vi "Measurement Logic.vi"() -> ()   [LabVIEW 2021, in "Single Tone Power Sweep.lvlib"]
uses:
  Single Tone Power Sweep.lvlib
  Measurement Configuration.ctl
  shared/controls/digital output level units.ctl
  shared/controls/weighting filter.ctl
  shared/controls/highpass filter.ctl
  shared/controls/lowpass filter.ctl
  shared/controls/units - snr.ctl
  shared/controls/units - ratio.ctl
  shared/controls/power measurement method.ctl
  Measurement Results.ctl
  <vilib>/MeasurementLink/MeasurementLink Measurement Server/Measure Call Context/Measure Call Context.lvclass
  <instrlib>/niDCPower/nidcpower.llb/niDCPower Source Mode.ctl
  <instrlib>/niDCPower/nidcpower.llb/niDCPower Output Function.ctl
  <instrlib>/niDMM/nidmm.llb/niDMM Function.ctl
  <instrlib>/niDMM/nidmm.llb/niDMM Resolution in Digits.ctl
  <vilib>/Analysis/1siggen.llb/Ramp Pattern by Samples.vi
  <instrlib>/niDMM/nidmm.llb/niDMM Configure Measurement Digits.vi
  <vilib>/Analysis/NI_AALBase.lvlib
  shared/controls/audio controls.lvlib
panel:
  out "XY Graph":cluster{"Array":dbl[], "Array":dbl[]}(graph)
  out "Spectrum":cluster{"x0":dbl, "dx":dbl, "magnitude":dbl[]}[](graph)
  out "Waveform Graph":waveform(dbl)[](graph)
  out "measure call context out":refnum<class "Measure Call Context.lvclass">
  in  "measure call context in":refnum<class "Measure Call Context.lvclass">
  out "measurement results":T1={"channel names"=[], "SNR"=[], "THD+N"=[], "THD"=[], "power supply voltage (V)"=[], "power supply current (A)"=[], "input power (W)"=[], "total output power (W)"=[], "power loss (W)"=[], "efficiency (%)"=[], "wfm - t0"=0.0, "wfm - dt"=1.9531249997269942e-05, "wfm - data"=array[12800 elements], "fft - f0"=0.0, "fft - df"=4.000000000559116, "fft - data"=array[6400 elements]}
  in  "measurement configuration":T2={"digital serial cfg file"="", "digital channel list"="7821\\PCMo 8", "master clock channel list"="7821\\PCMo 0", "output level start"=10.0, "output level stop"=60.0, "output sweep number of steps"=5, "output level units"=enum."% FS", "output range (pk-pk)"=15.0, "load impedance"=4.0, "signal phase"=0.0, "acq sampling rate"=51200.0, "min measurement cycles"=20, "min measurement time (s)"=0.1, "min settling cycles"=0, "min settling time (s)"=0.005, "acq channel"="PXI1Slot4/ai0", "band start"=20.0, "band stop"=20000.0, "weighting filter"=enum."Linear", "highpass filter"=enum."DC", "lowpass filter"=enum."No filter", "SNR units"=enum."dB", "THD+N units"=enum."dB", "THD units"=enum."dB", "gain units"=enum."dB", "power measurement method"=enum."DMM", "power measurement resource"="PXI1Slot9", "power supply voltage"=14.4, "power supply current limit"=1.2, "sense resistor (Ohms)"=0.01} {"band start" format="%0.2f"; "acq sampling rate" format="%0.2f"; "signal phase" format="%#_6p"}
  out "error out":errorcluster
  in  "error in":errorcluster
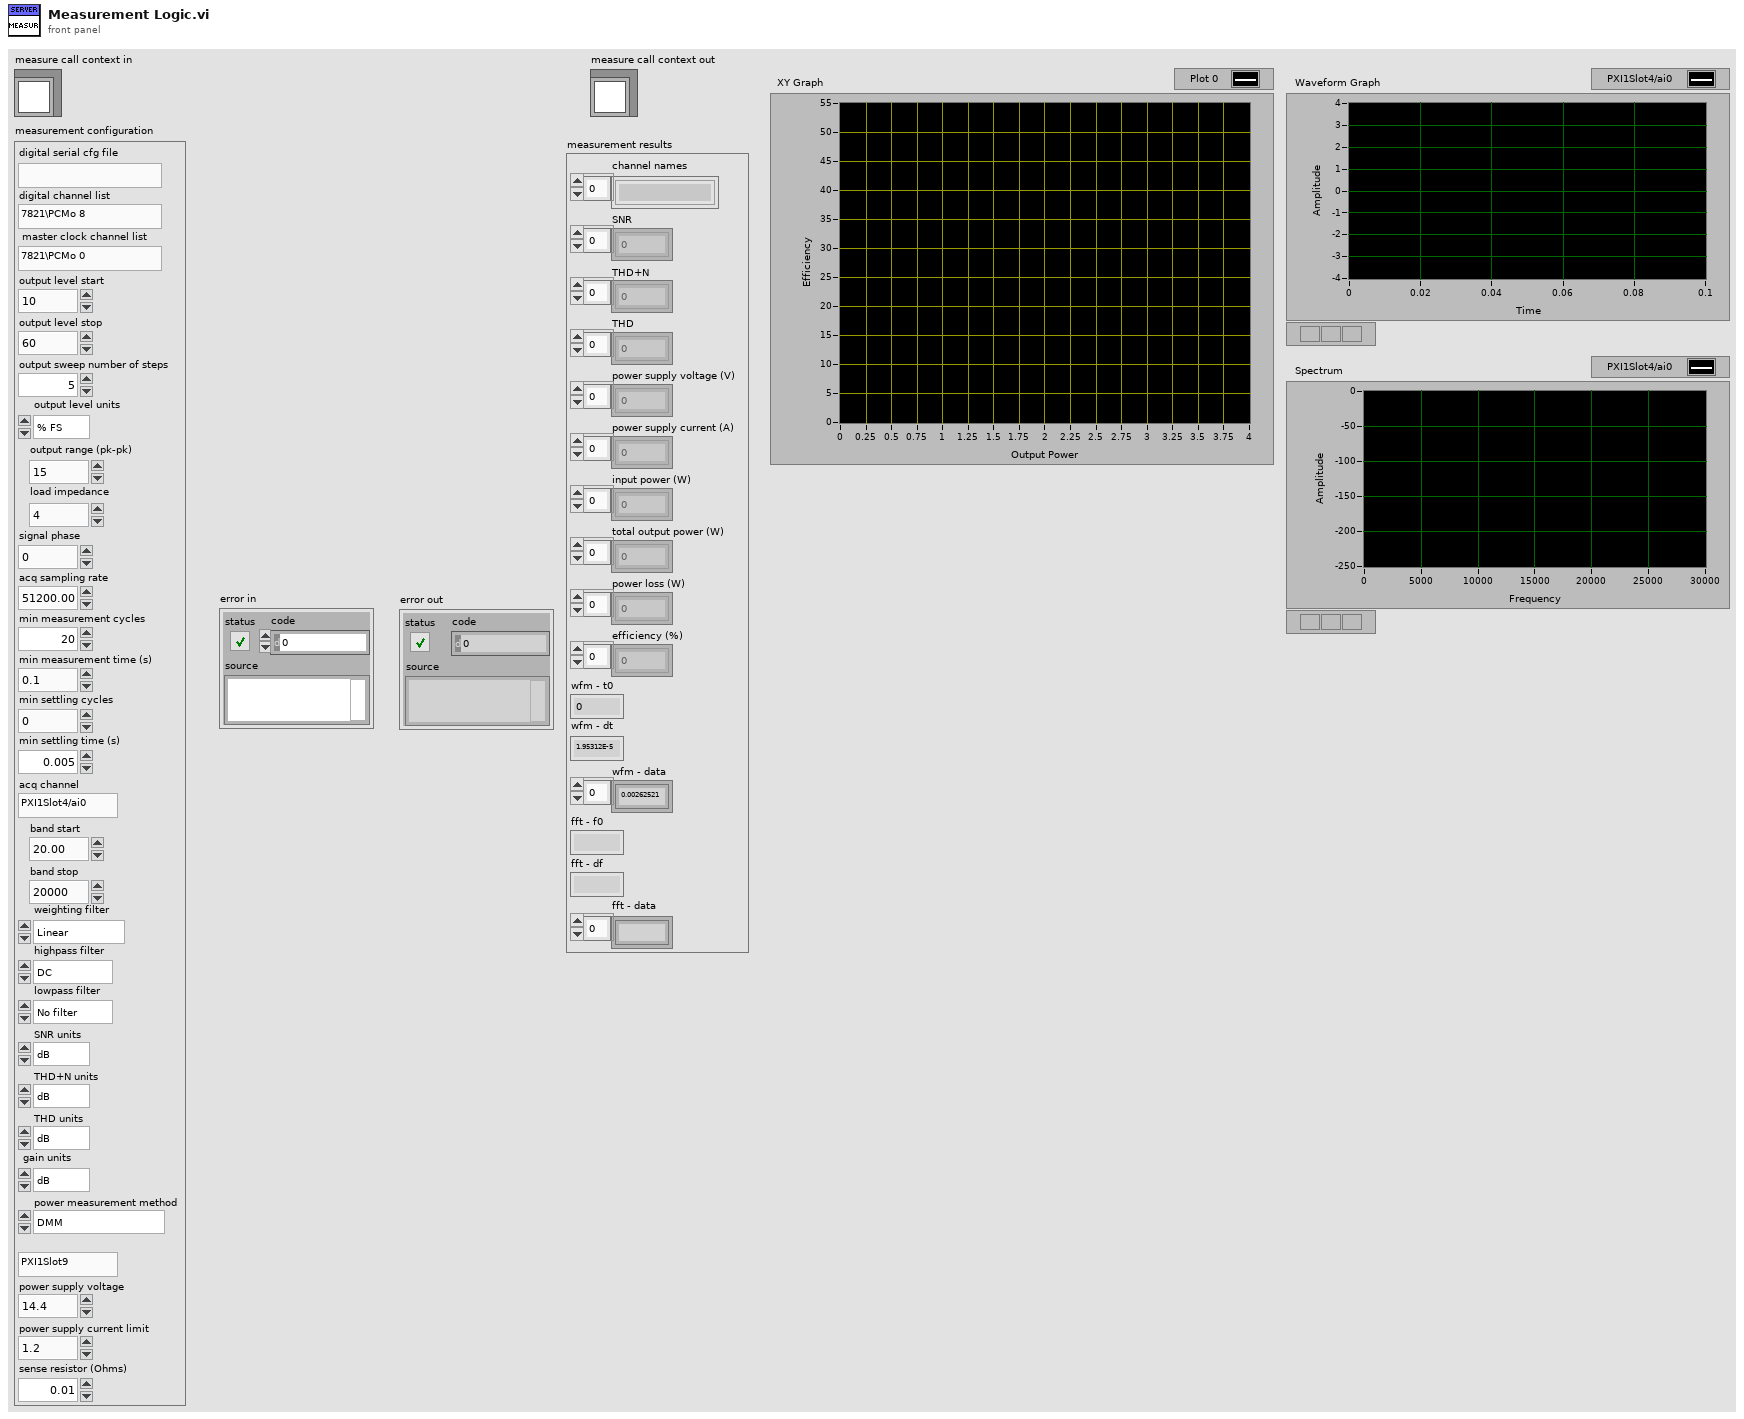
[diagram p1: front panel]
types:
  T1 = typedef "Single Tone Power Sweep.lvlib/Measurement Results.ctl" = cluster{"channel names":string[], "SNR":dbl[], "THD+N":dbl[], "THD":dbl[], "power supply voltage (V)":dbl[], "power supply current (A)":dbl[], "input power (W)":dbl[], "total output power (W)":dbl[], "power loss (W)":dbl[], "efficiency (%)":dbl[], "wfm - t0":dbl, "wfm - dt":dbl, "wfm - data":dbl[], "fft - f0":dbl, "fft - df":dbl, "fft - data":dbl[]}
  T2 = typedef "Single Tone Power Sweep.lvlib/Measurement Configuration.ctl" = cluster{"digital serial cfg file":string, "digital channel list":string, "master clock channel list":string, "output level start":dbl, "output level stop":dbl, "output sweep number of steps":u32, "output level units":T3, "output range (pk-pk)":dbl, "load impedance":dbl, "signal phase":dbl, "acq sampling rate":dbl, "min measurement cycles":u32, "min measurement time (s)":dbl, "min settling cycles":u32, "min settling time (s)":dbl, "acq channel":string, "band start":dbl, "band stop":dbl, "weighting filter":T4, "highpass filter":T5, "lowpass filter":T6, "SNR units":T7, "THD+N units":T8, "THD units":T8, "gain units":T8, "power measurement method":T9, "power measurement resource":string, "power supply voltage":dbl, "power supply current limit":dbl, "sense resistor (Ohms)":dbl}
  T3 = typedef "audio controls.lvlib/digital output level units.ctl" = enum32{"% FS", "dBFS", "V"}
  T4 = typedef "weighting filter.ctl" = enum32{"Linear", "A-weighting", "B-weighting", "C-weighting"}
  T5 = typedef "highpass filter.ctl" = enum32{"DC", "AC"}
  T6 = typedef "lowpass filter.ctl" = enum32{"No filter", "AES17 20kHz", "AES17 40kHz"}
  T7 = typedef "audio controls.lvlib/units - snr.ctl" = enum32{"dB", "x/y"}
  T8 = typedef "audio controls.lvlib/units - ratio.ctl" = enum32{"dB", "%", "x/y"}
  T9 = typedef "power measurement method.ctl" = enum32{"SMU", "DMM"}
  T10 = typedef "niDMM Function.ctl" = enum16{"DC Volts", "AC Volts", "DC Current", "AC Current", "2-wire Resistance", "4-wire Resistance", "Diode", "Frequency", "Period", "AC Volts DC Coupled", "Capacitance", "Inductance", "Temperature"}
  T11 = typedef "niDCPower Output Function.ctl" = i32
  T12 = typedef "niDCPower Source Mode.ctl" = i32
  T13 = typedef "niDMM Resolution in Digits.ctl" = dbl
  T14 = typedef "single tone measurement settings (HW).ctl" = cluster{"digital channel list":string, "frame clock rate":dbl, "number of channels":u32, "channel length":u32, "bit depth":u32, "data justification":T15, "endianness":T16, "bit clock edge sync":T17, "frame sync edge for channel 0":T17, "channel 0 offset":u32, "master clock channel list":string, "master clock rate":dbl, "enable dither":bool, "logic level":T18, "signal frequency":dbl, "output level":dbl, "output level units":T3, "output range (pk-pk)":dbl, "load impedance":dbl, "signal phase":dbl, "acq sampling rate":dbl, "min measurement cycles":u32, "min measurement time (s)":dbl, "min settling cycles":u32, "min settling time (s)":dbl, "acq channel":string, "band start":dbl, "band stop":dbl, "weighting filter":T4, "highpass filter":T5, "lowpass filter":T6, "SNR units":T7, "THD+N units":T8, "THD units":T8, "gain units":T8}
  T15 = typedef "data justification.ctl" = enum32{"Left Justified", "Right Justified"}
  T16 = typedef "endianness.ctl" = enum32{"MSB First", "LSB First"}
  T17 = typedef "digital edge.ctl" = enum32{"Rising", "Falling"}
  T18 = typedef "logic level.ctl" = enum32{"3.3 V", "1.8 V", "1.2 V"}
  T19 = typedef "PCM tasks.ctl" = cluster{"PCM output task":T20, "PCM output task-clock":T20}
  T20 = typedef "PDM Acquisition Class Library.lvlib/PCM Output Task.lvclass/PCM Output Task DVR.ctl" = refnum<data-value>
  T21 = typedef "audio controls.lvlib/single tone audio measurements.ctl" = cluster{"channel":string, "frequency (Hz)":dbl, "amplitude (Vrms)":dbl, "amplitude (dBFS)":dbl, "phase (deg)":dbl, "SNR":dbl, "THD+N":dbl, "THD":dbl, "dynamic range (dB)":dbl, "gain":dbl, "SFDR (dBc)":dbl}
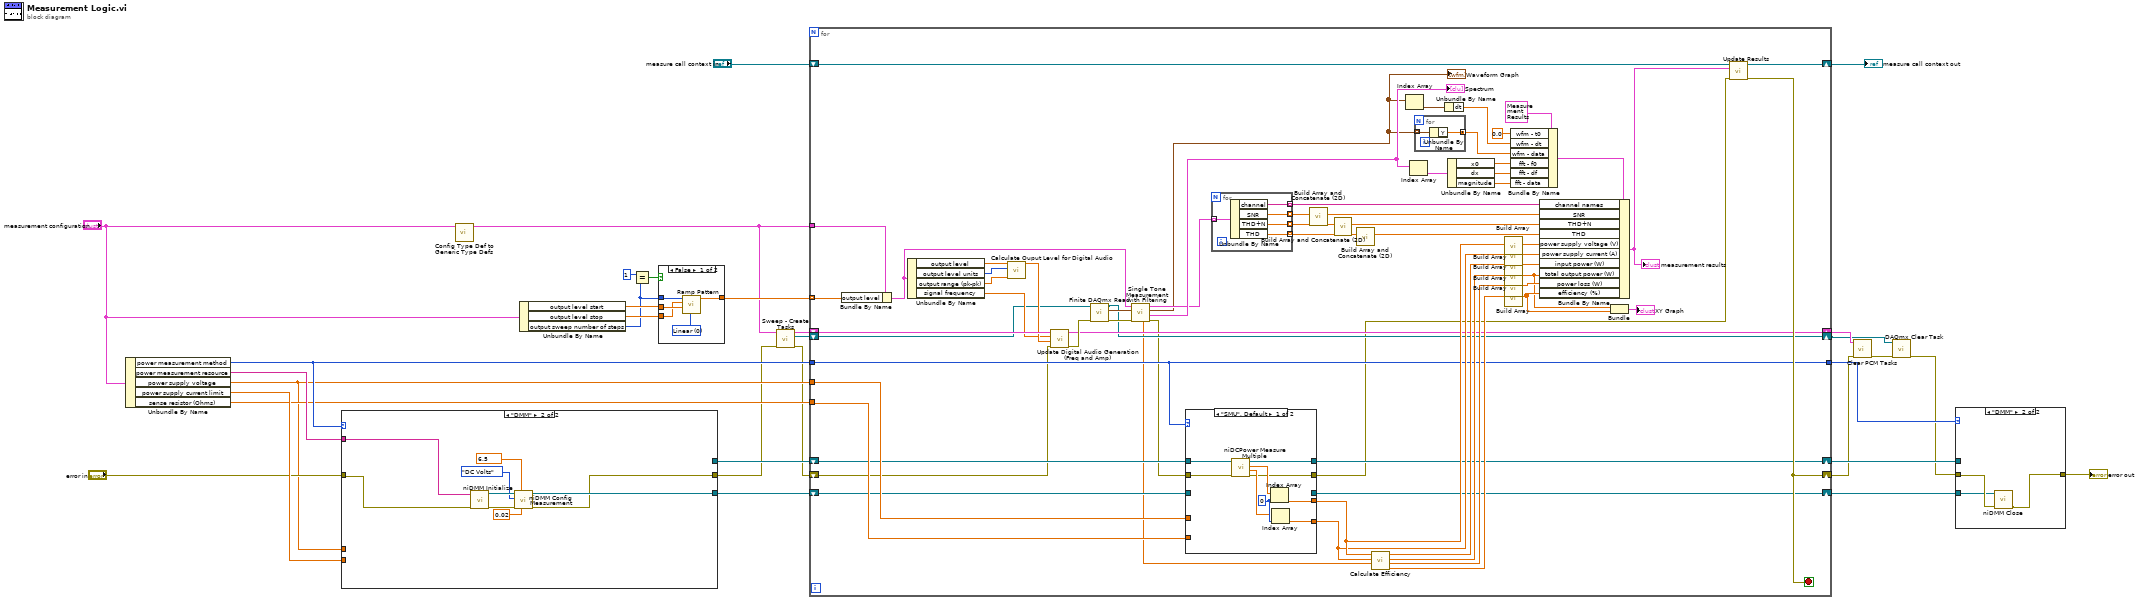
[diagram p0: block diagram]
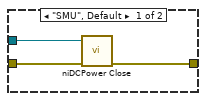
[diagram p2: hidden frame]
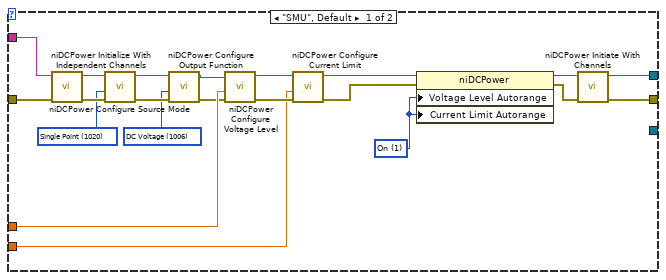
[diagram p3: hidden frame]
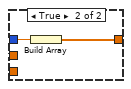
[diagram p4: hidden frame]
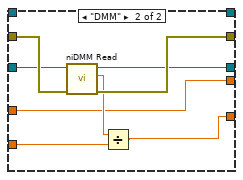
[diagram p5: hidden frame]
diagram:
  n1 = Unbundle By Name("measurement configuration") -> ("power measurement method"=w20:T9, "power measurement resource"=w23:string, "power supply voltage"=w18:dbl, "power supply current limit"=w22:dbl, "sense resistor (Ohms)"=w19:dbl)
  n2 = case shown="\"DMM\"" w20 {
    tunnel: w18 -> [w50 _]
    tunnel: w22 -> [w49 _]
    tunnel: [w35 _] -> w11
    tunnel: [w34 w57] -> w10
    tunnel: "error in" -> [w33 w61]
    tunnel: [_ w58] -> w12
    tunnel: w23 -> [w32 w53]
    frame "SMU", Default {
      w36 = 1 items=["Off", "On"] ("Source:DC Voltage:Current Limit Autorange")
      w37 = T11 1006 items=["DC Voltage"=1006, "DC Current"=1007, "Pulse Voltage"=1049, "Pulse Current"=1050] ("output function")
      w44 = T12 1020 items=["Single Point"=1020, "Sequence"=1021] ("source mode")
      n3 = call <instrlib>:"niDCPower Initialize With Independent Channels.vi"("error in (no error)"=w33, "resource name"=w32) -> ("error out"=w48:errorcluster, "instrument handle out"=w47:refnum<k15>)  [unwired: 8 in]
      n4 = call <instrlib>:"niDCPower Configure Source Mode.vi"("error in (no error)"=w48, "source mode"=w44, "instrument handle"=w47) -> ("error out"=w46:errorcluster, "instrument handle out"=w45:refnum<k15>)  [unwired: 7 out]
      n5 = call <instrlib>:"niDCPower Configure Output Function.vi"("error in (no error)"=w46, "output function"=w37, "instrument handle"=w45) -> ("error out"=w38:errorcluster, "instrument handle out"=w39:refnum<k15>)  [unwired: 1 in, 6 out]
      n6 = call <instrlib>:"niDCPower Configure Voltage Level.vi"("error in (no error)"=w38, "voltage level"=w50, "instrument handle"=w39) -> ("error out"=w51:errorcluster, "instrument handle out"=w52:refnum<k15>)  [unwired: 1 in, 6 out]
      n7 = call <instrlib>:"niDCPower Configure Current Limit.vi"("error in (no error)"=w51, "current limit"=w49, "instrument handle"=w52) -> ("error out"=w40:errorcluster, "instrument handle out"=w43:refnum<k15>)  [unwired: 2 in, 5 out]
      n8 = property class="niDCPower"(reference=w43, error in=w40, "Voltage Level Autorange"=w36, "Current Limit Autorange"=w36) -> (reference out=w42:refnum<k15>, error out=w41:errorcluster)
      n9 = call <instrlib>:"niDCPower Initiate With Channels.vi"("error in (no error)"=w41, "instrument handle"=w42) -> ("error out"=w34:errorcluster, "instrument handle out"=w35:refnum<k15>)  [unwired: 8 in]
    }
    frame "DMM" {
      w55 = T13 6.5 items=["3 1/2"=3.5, "4 1/2"=4.5, "5 1/2"=5.5, "6 1/2"=6.5, "7 1/2"=7.5] ("Resolution in Digits")
      n10 = call <instrlib>:"niDMM Initialize.vi"("error in (no error)"=w61, "Instrument Descriptor"=w53) -> ("error out"=w60:errorcluster, "instrument handle out"=w59:refnum<k15>)  [unwired: 8 in]
      n11 = call-poly <instrlib>:"niDMM Config Measurement.vi"("Range"=0.02, "Resolution in Digits"=w55, "error in (no error)"=w60, "Function"=niDMM_Function."DC Volts", "instrument handle"=w59) -> ("error out"=w57:errorcluster, "instrument handle out"=w58:refnum<k15>)  [unwired: 5 in]
    }
  }
  n12 = call "Config Type Def to Generic Type Defs.vi"("measurement configuration"="measurement configuration") -> ("single tone settings"=w9:T14)  [unwired: 9 in, 1 out]
  n13 = Unbundle By Name("measurement configuration") -> ("output level start"=w31:dbl, "output level stop"=w30:dbl, "output sweep number of steps"=w26:u32)
  n14 = Equal?(x=u32 1, y=w26) -> (x = y?=w27:bool)
  n15 = case shown="False" w27 {
    tunnel: w31 -> [w66 w68]
    tunnel: w30 -> [w65 _]
    tunnel: w26 -> [w64 _]
    tunnel: [w63 w67] -> w29
    frame False {
      w62 = u16 0 items=["Linear", "Logarithmic"] ("type")
      n16 = call-poly <vilib>:"Ramp Pattern.vi"("type"=w62, "start"=w66, "end"=w65, "samples"=w64) -> ("Ramp Pattern"=w63:dbl[])  [unwired: 6 in, 1 out]
    }
    frame True {
      n17 = Build Array(w68) -> (w67:dbl[])
    }
  }
  n18 = call "Sweep - Create Tasks.vi"("error in (no error)"=w10, "measurement configuration"=w9) -> ("error out"=w6:errorcluster, "DAQmx task"=w7:refnum<k21>, "PCM tasks"=w8:T19)  [unwired: 7 in]
  n19 = for {
    tunnel: w29 -> [w106] mode=indexing
    shift-right: [w105] -> w2
    shift-left: w6 -> [w81]
    shift-right: [w131] -> w28
    shift-left: "measure call context in" -> [w130]
    tunnel: w20 -> [w104]
    tunnel: w19 -> [w121]
    tunnel: w18 -> [w120]
    tunnel: w9 -> [w107]
    tunnel: [w104] -> w15
    shift-right: [w103] -> w14
    shift-left: w11 -> [w97]
    shift-right: [w102] -> w13
    shift-left: w12 -> [w98]
    shift-right: [w89] -> w4
    shift-left: w8 -> [w90]
    shift-right: [w85] -> w3
    shift-left: w7 -> [w84]
    stop <- w105 stop-if-true
    n20 = Bundle By Name(cluster=w107, "output level"=w106) -> (w86:T14)
    n21 = Unbundle By Name(w86) -> ("output level"=w96:dbl, "output level units"=w95:T3, "output range (pk-pk)"=w94:dbl, "signal frequency"=w87:dbl)
    n22 = call "Calculate Ouput Level for Digital Audio.vi"("output range (pk-pk)"=w94, "digital output level units"=w95, "output level"=w96) -> ("gain"=w88:dbl)  [unwired: 7 in, 1 out]
    n23 = call "Update Digital Audio Generation (Freq and Amp).vi"("error in (no error)"=w81, "gain"=w88, "frequency"=w87, "PCM tasks"=w90) -> ("error out"=w93:errorcluster, "PCM tasks"=w89:T19)  [unwired: 6 in]
    n24 = call "Finite DAQmx Read.vi"("error in (no error)"=w93, "task/channels in"=w84) -> ("error out"=w92:errorcluster, "data"=w91:waveform(dbl)[], "task out"=w85:refnum<k21>)  [unwired: 7 in]
    n25 = call "Single Tone Measurement with Filtering.vi"("error in (no error)"=w92, "waveforms"=w91, "measurement configuration"=w86) -> ("error out"=w83:errorcluster, "spectra"=w79:cluster{"x0":dbl, "dx":dbl, "magnitude":dbl[]}[], "waveforms"=w70:waveform(dbl)[], "results"=w78:T21[], "output power"=w80:dbl[])  [unwired: 4 in]
    "Waveform Graph" <- w70
    "Spectrum" <- w79
    n26 = case shown="\"SMU\", Default" w104 {
      tunnel: [w147 _] -> w103
      tunnel: [w146 w148] -> w115
      tunnel: [w145 w152] -> w114
      tunnel: [w141 w154] -> w82
      tunnel: w83 -> [w140 w155]
      tunnel: [_ w151] -> w102
      tunnel: w98 -> [_ w150]
      tunnel: w97 -> [w139 _]
      tunnel: w121 -> [_ w149]
      tunnel: w120 -> [_ w148]
      frame "SMU", Default {
        w144 = 0 ("index")
        n27 = call <instrlib>:"niDCPower Measure Multiple.vi"("error in (no error)"=w140, "instrument handle"=w139) -> ("error out"=w141:errorcluster, "current measurements"=w142:dbl[], "voltage measurements"=w143:dbl[], "instrument handle out"=w147:refnum<k15>)  [unwired: 6 in]
        n28 = Index Array(array=w143, index=w144) -> (element=w146:dbl)
        n29 = Index Array(array=w142, index=w144) -> (element=w145:dbl)
      }
      frame "DMM" {
        n30 = call <instrlib>:"niDMM Read.vi"("error in (no error)"=w155, "instrument handle"=w150) -> ("error out"=w154:errorcluster, "Measurement"=w153:dbl, "instrument handle out"=w151:refnum<k15>)  [unwired: 7 in]
        n31 = Divide(x=w153, y=w149) -> (x/y=w152:dbl)
      }
    }
    n32 = for {
      tunnel: w78 -> [w138] mode=indexing
      tunnel: [w137] -> w77 mode=indexing
      tunnel: [w136] -> w76 mode=indexing
      tunnel: [w135] -> w74 mode=indexing
      tunnel: [w134] -> w72 mode=indexing
      n33 = Unbundle By Name(w138) -> ("channel"=w137:string, "SNR"=w136:dbl, "THD+N"=w135:dbl, "THD"=w134:dbl)
    }
    n34 = call "Build Array and Concatenate (2D).vi"("Array"=w76) -> ("Array Out"=w75:dbl[])  [unwired: 10 in]
    n35 = call "Build Array and Concatenate (2D).vi"("Array"=w74) -> ("Array Out"=w73:dbl[])  [unwired: 10 in]
    n36 = call "Build Array and Concatenate (2D).vi"("Array"=w72) -> ("Array Out"=w71:dbl[])  [unwired: 10 in]
    n37 = call "Calculate Efficiency.vi"("output power per channel"=w80, "power supply current"=w114, "power supply voltage"=w115) -> ("efficiency"=w110:dbl, "power loss"=w111:dbl, "total output power"=w112:dbl, "input power"=w113:dbl)  [unwired: 5 in]
    n38 = Index Array(array=w70) -> (element=w109:waveform(dbl))  [unwired: 1 in]
    n39 = Index Array(array=w79) -> (element=w108:cluster{"x0":dbl, "dx":dbl, "magnitude":dbl[]})  [unwired: 1 in]
    n40 = for {
      tunnel: w70 -> [w133] mode=indexing
      tunnel: [w132] -> w69 mode=concatenating
      n41 = Unbundle By Name(w133) -> ("Y"=w132:dbl[])
    }
    n42 = Unbundle By Name(w109) -> ("dt"=w125:dbl)
    n43 = Unbundle By Name(w108) -> ("x0"=w124:dbl, "dx"=w123:dbl, "magnitude"=w122:dbl[])
    n44 = call "Build Array.vi"("value"=w115) -> ("Array"=w119:dbl[])  [unwired: 10 in]
    n45 = call "Build Array.vi"("value"=w114) -> ("Array"=w118:dbl[])  [unwired: 10 in]
    n46 = call "Build Array.vi"("value"=w113) -> ("Array"=w117:dbl[])  [unwired: 10 in]
    n47 = call "Build Array.vi"("value"=w112) -> ("Array"=w100:dbl[])  [unwired: 10 in]
    n48 = call "Build Array.vi"("value"=w111) -> ("Array"=w116:dbl[])  [unwired: 10 in]
    n49 = call "Build Array.vi"("value"=w110) -> ("Array"=w101:dbl[])  [unwired: 10 in]
    n50 = Bundle By Name(cluster=T1 {"channel names"=[], "SNR"=[], "THD+N"=[], "THD"=[], "power supply voltage (V)"=[], "power supply current (A)"=[], "input power (W)"=[], "total output power (W)"=[], "power loss (W)"=[], "efficiency (%)"=[], "wfm - t0"=0.0, "wfm - dt"=0.0, "wfm - data"=[], "fft - f0"=0.0, "fft - df"=0.0, "fft - data"=[]} ("Measurement Results"), "wfm - t0"=0.0, "wfm - dt"=w125, "wfm - data"=w69, "fft - f0"=w124, "fft - df"=w123, "fft - data"=w122) -> (w127:T1)
    n51 = Bundle By Name(cluster=w127, "channel names"=w77, "SNR"=w75, "THD+N"=w73, "THD"=w71, "power supply voltage (V)"=w119, "power supply current (A)"=w118, "input power (W)"=w117, "total output power (W)"=w100, "power loss (W)"=w116, "efficiency (%)"=w101) -> (w126:T1)
    "measurement results" <- w126
    n52 = Bundle("Array"=w100, "Array"=w101) -> (→"XY Graph":cluster{"Array":dbl[], "Array":dbl[]})  [unwired: 1 in]
    n53 = call <vilib>:"Update Results.vi"("error in"=w82, "measurement results"=w126, "measure call context in"=w130) -> ("error out"=w105:errorcluster, "measure call context out"=w131:refnum<class "Measure Call Context.lvclass">)  [unwired: 7 in]
  }
  "measure call context out" <- w28
  n54 = call "Clear PCM Tasks.vi"("error in (no error)"=w2, "PCM tasks"=w4) -> ("error out"=w5:errorcluster)  [unwired: 9 in]
  n55 = call <vilib>:"DAQmx Clear Task.vi"("task in"=w3, "error in"=w5) -> ("error out"=w1:errorcluster)  [unwired: 13 in]
  n56 = case shown="\"DMM\"" w15 {
    tunnel: [w158 w160] -> w16
    tunnel: w1 -> [w157 w161]
    tunnel: w14 -> [w156 _]
    tunnel: w13 -> [_ w159]
    frame "SMU", Default {
      n57 = call <instrlib>:"niDCPower Close.vi"("error in (no error)"=w157, "instrument handle"=w156) -> ("error out"=w158:errorcluster)  [unwired: 9 out]
    }
    frame "DMM" {
      n58 = call <instrlib>:"niDMM Close.vi"("error in (no error)"=w161, "instrument handle"=w159) -> ("error out"=w160:errorcluster)  [unwired: 9 in]
    }
  }
  "error out" <- w16
